vi "Move WindowTopLeft to MousePointer location.vi"(8 "error in (no error)":errorcluster, 11 "VIRef":refnum<vi>) -> (0 "error out":errorcluster)   [LabVIEW 2017]
uses:
  <vilib>/Utility/inputDevices.llb/closeMouse.vi
  <vilib>/Utility/inputDevices.llb/mouseAcquire.vi
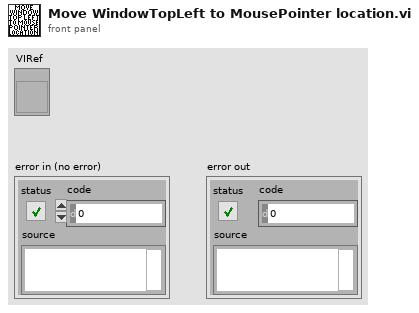
[diagram p1: front panel]
types:
  T1 = cluster{"Horizontal":i32, "Vertical":i32, "Scrolling":i32}
  T2 = typedef "LVRectTypeDef.ctl" = cluster{"Left":i16, "Top":i16, "Right":i16, "Bottom":i16}
  T3 = cluster{"Horizontal":i16, "Vertical":i16, "Scrolling":i16}
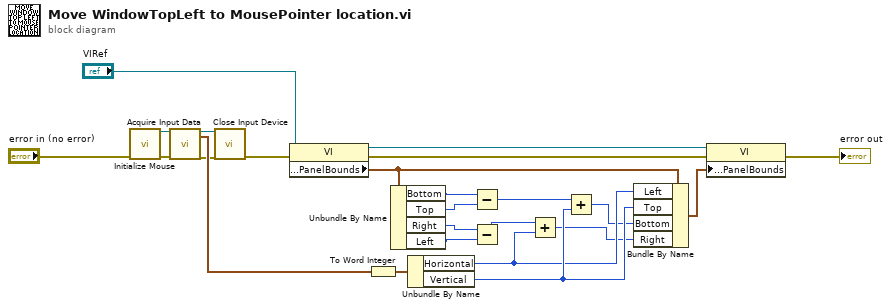
[diagram p0: block diagram]
diagram:
  n1 = call <vilib>:"Initialize Mouse.vi"("error in (no error)"="error in (no error)") -> ("error out"=w2:errorcluster, "device ID"=w3:refnum<k1>)  [unwired: 9 in]
  n2 = call-poly <vilib>:"Acquire Input Data.vi"("device ID"=w3, "error in (no error)"=w2) -> ("device ID"=w5:refnum<k1>, "axis info"=w6:T1, "error out"=w4:errorcluster)  [unwired: 14 in, 1 out]
  n3 = call-poly <vilib>:"Close Input Device.vi"("error in (no error)"=w4, "device ID"=w5) -> ("error out"=w17:errorcluster)  [unwired: 8 in]
  n4 = property class="VI"(reference="VIRef", error in=w17) -> (reference out=w24:refnum<vi>, error out=w16:errorcluster, "Front Panel.PanelBounds"=w8:T2)
  n5 = To Word Integer(number=w6) -> (16bit integer=w13:T3)
  n6 = Unbundle By Name(w8) -> ("Bottom"=w9:i16, "Top"=w10:i16, "Right"=w11:i16, "Left"=w12:i16)
  n7 = Unbundle By Name(w13) -> ("Horizontal"=w20:i16, "Vertical"=w21:i16)
  n8 = Subtract(x=w9, y=w10) -> (x-y=w18:i16)
  n9 = Subtract(x=w11, y=w12) -> (x-y=w19:i16)
  n10 = Add(x=w19, y=w20) -> (x+y=w15:i16)
  n11 = Add(x=w18, y=w21) -> (x+y=w14:i16)
  n12 = Bundle By Name(cluster=w8, "Left"=w20, "Top"=w21, "Bottom"=w14, "Right"=w15) -> (w7:T2)
  n13 = property class="VI"(reference=w24, error in=w16, "Front Panel.PanelBounds"=w7) -> (error out=→"error out":errorcluster)  [unwired: 1 out]
